vi "ElevatorNetwork.vi"(8 "error in (no error)":errorcluster) -> (0 "error out":errorcluster)   [LabVIEW 2023]
uses:
  <vilib>/Rock Robotics/Network Tables/NT Write Boolean.vi
  ElevatorGlobal.vi
  <vilib>/Rock Robotics/Network Tables/NT Write Number.vi
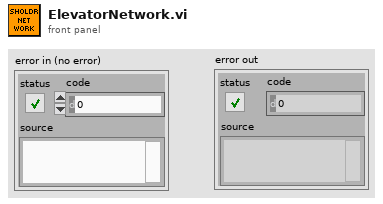
[diagram p1: front panel]
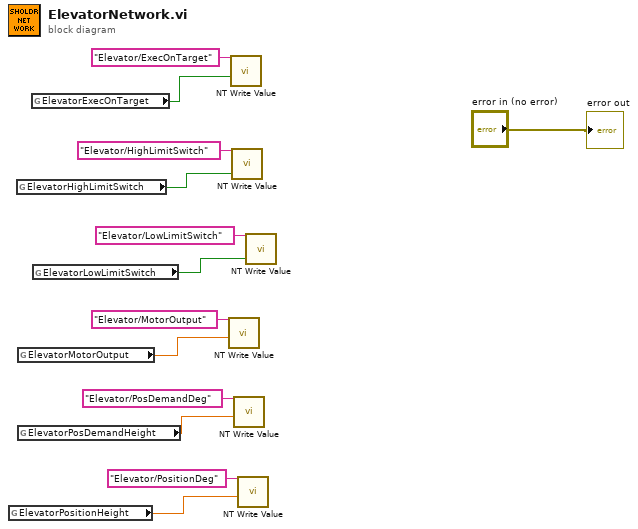
[diagram p0: block diagram]
diagram:
  n1 = global read "ElevatorGlobal.vi" "ElevatorPositionHeight"() -> (w7:dbl)
  n2 = global read "ElevatorGlobal.vi" "ElevatorHighLimitSwitch"() -> (w4:bool)
  n3 = global read "ElevatorGlobal.vi" "ElevatorMotorOutput"() -> (w5:dbl)
  n4 = global read "ElevatorGlobal.vi" "ElevatorPosDemandHeight"() -> (w6:dbl)
  n5 = global read "ElevatorGlobal.vi" "ElevatorExecOnTarget"() -> (w3:bool)
  n6 = global read "ElevatorGlobal.vi" "ElevatorLowLimitSwitch"() -> (w1:bool)
  n7 = call-poly <vilib>:"NT Write Value.vi"("value"=w5, "name"="Elevator/MotorOutput") -> ()  [unwired: 9 in, 1 out]
  n8 = call-poly <vilib>:"NT Write Value.vi"("value"=w3, "name"="Elevator/ExecOnTarget") -> ()  [unwired: 9 in, 1 out]
  n9 = call-poly <vilib>:"NT Write Value.vi"("value"=w4, "name"="Elevator/HighLimitSwitch") -> ()  [unwired: 9 in, 1 out]
  n10 = call-poly <vilib>:"NT Write Value.vi"("value"=w6, "name"="Elevator/PosDemandDeg") -> ()  [unwired: 9 in, 1 out]
  n11 = call-poly <vilib>:"NT Write Value.vi"("value"=w7, "name"="Elevator/PositionDeg") -> ()  [unwired: 9 in, 1 out]
  n12 = call-poly <vilib>:"NT Write Value.vi"("value"=w1, "name"="Elevator/LowLimitSwitch") -> ()  [unwired: 9 in, 1 out]
  "error out" <- "error in (no error)"
